vi "LVClass_WavefrontCorrector Set Temporization.vi"(0 "WavefrontCorrector in":refnum<class "WavefrontCorrector.lvclass">, 5 "Sleep after command apply (ms)":i32, 11 "error in (no error)":errorcluster) -> (4 "WavefrontCorrector out":refnum<class "WavefrontCorrector.lvclass">, 15 "error out":errorcluster)   [LabVIEW 2020, in "WavefrontCorrector.lvclass"]
uses:
  WavefrontCorrector.lvclass
  WavefrontCorrector.lvclass/WavefrontCorrector.ctl
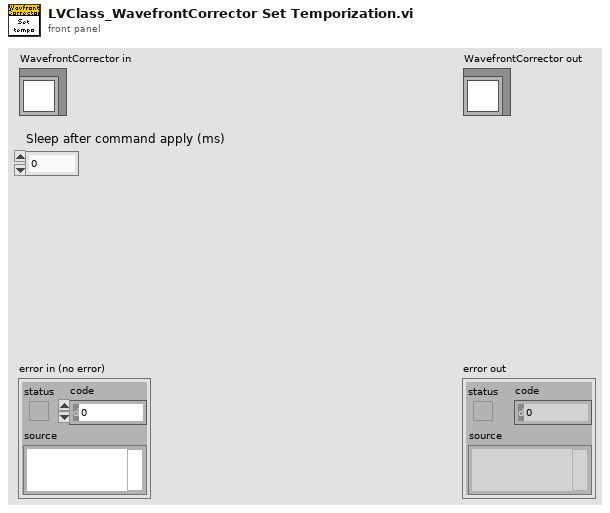
[diagram p1: front panel]
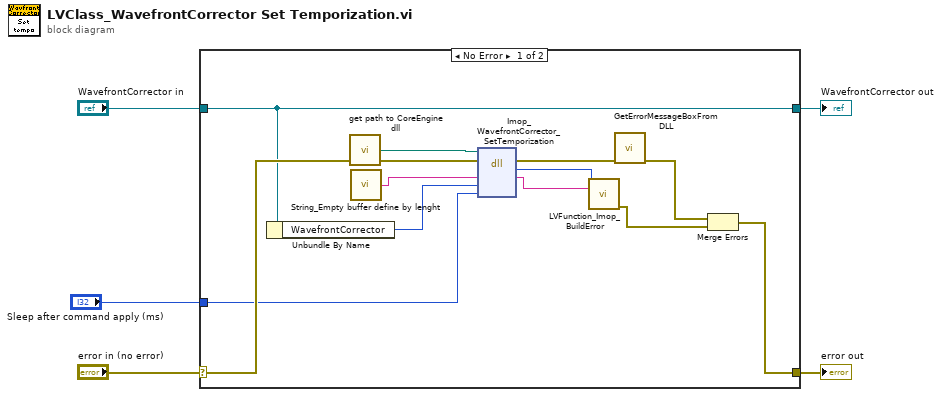
[diagram p0: block diagram]
diagram:
  n1 = case shown="No Error" "error in (no error)" {
    selector: "error in (no error)" -> [w15 w19]
    tunnel: [w6 w19] -> w4
    tunnel: [w14 w18] -> w2
    tunnel: "WavefrontCorrector in" -> [w14 w18]
    tunnel: "Sleep after command apply (ms)" -> [w12 _]
    frame No Error {
      n2 = Unbundle By Name(w14) -> ("WavefrontCorrector"=w13:i32)
      n3 = call "get path to CoreEngine dll.vi"() -> ("path to c_interface_vc100.dll"=w17:path)  [unwired: 12 in, 3 out]
      n4 = call "String_Empty buffer define by lenght.vi"() -> ("Empty buffer"=w16:string)  [unwired: 1 in]
      n5 = dll-call lib="D:/FLE/0.Code/CoreEngine4_Suite/LV2011_interface/DLLs/c_interface_vc100.dll" fn="Imop_WavefrontCorrector_SetTemporization"(path in=w17, error in=w15, "message"=w16, "WavefrontCorrector"=w13, "Sleep after movement"=w12) -> (error out=w9:errorcluster, "return type"=w11:i32, "message"=w10:string)  [unwired: 3 in, 1 out]
      n6 = call "LVFunction_Imop_BuildError.vi"("code"=w11, "String to Prepend to source (\"\")"=w10) -> ("error out"=w7:errorcluster)  [unwired: 13 in]
      n7 = call "GetErrorMessageBoxFromDLL.vi"("error IN"=w9) -> ("error OUT"=w8:errorcluster)  [unwired: 10 in]
      n8 = Merge Errors(w8, w7) -> (w6:errorcluster)
    }
    frame Error {
    }
  }
  "error out" <- w4
  "WavefrontCorrector out" <- w2
